vi "Index to cluster.vi"(8 "error in":errorcluster, 10 "Input Mapping Info":T1, 11 "Variant in":variant) -> (0 "error out":errorcluster, 3 "Variant out":variant)   [LabVIEW 2013]
uses:
  Channel Run Time Mapping Info.ctl
  <vilib>/Utility/VariantDataType/Type.ctl
  <vilib>/Utility/VariantDataType/VariantType.lvlib
  <vilib>/NI/Tag Bus Module Framework/root configuration/TBM configuration.lvclass
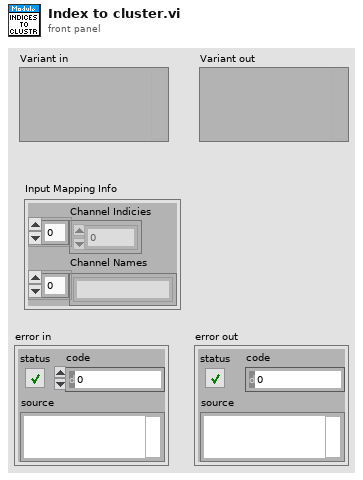
[diagram p1: front panel]
types:
  T1 = typedef "Channel Run Time Mapping Info.ctl" = cluster{"Channel Indicies":i32[], "Channel Names":string[]}
  T2 = typedef "VariantType.lvlib/Type.ctl" = enum8{"Invalid Type", "Void", "I8", "I16", "I32", "I64", "U8", "U16", "U32", "U64", "Single Float", "Double Float", "Extended Float", "Single Complex", "Double Complex", "Extended Complex", "Enum U8", "Enum U16", "Enum U32", "Enum U64", "Single Float With Unit", "Double Float With Unit", "Extended Float With Unit", "Single Complex with Unit", "Double Complex with Unit", "Extended Complex with Unit", "Boolean", "String", "Path", "Picture", "Tag", "Array", "Cluster", "Variant", "LV Variant", "Waveform", "Timestamp", "Digital Waveform", "Digital Data", "ExpressData", "Refnum", "External Data", "VI", "Poly VI", "LabVIEW Class Instance", "Fixed Point"}
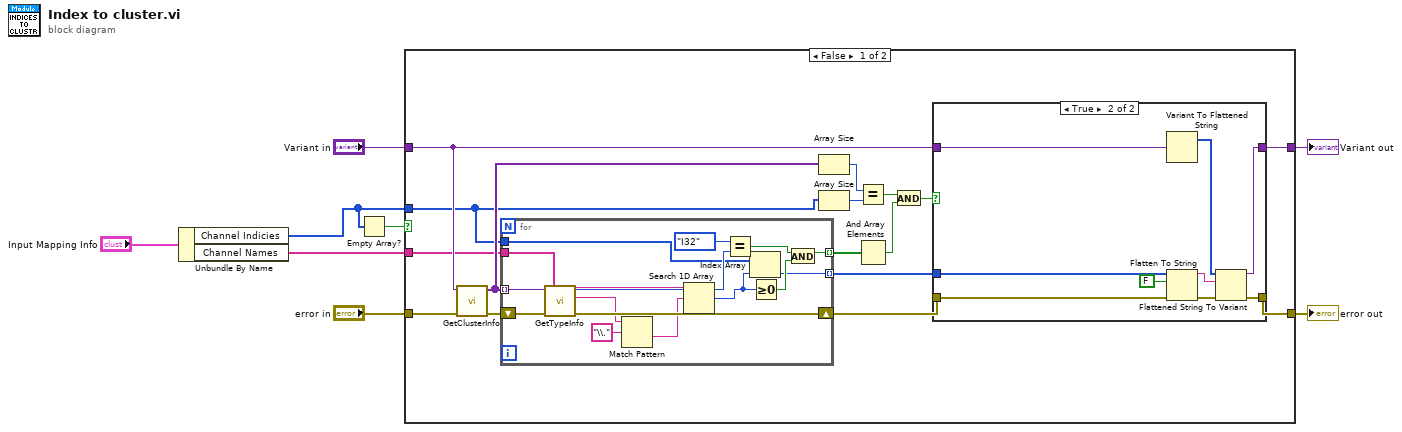
[diagram p0: block diagram]
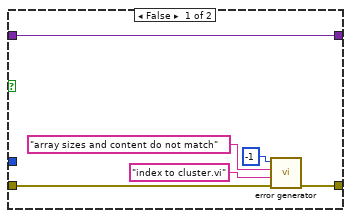
[diagram p2: hidden frame]
diagram:
  n1 = Unbundle By Name("Input Mapping Info") -> ("Channel Indicies"=w2:i32[], "Channel Names"=w1:string[])
  n2 = Empty Array?(array=w2) -> (empty?=w4:bool)
  n3 = case shown="False" w4 {
    tunnel: [w24 w56] -> w8
    tunnel: [w23 w55] -> w7
    tunnel: "error in" -> [w22 w55]
    tunnel: "Variant in" -> [w21 w56]
    tunnel: w2 -> [w10 _]
    tunnel: w1 -> [w11 _]
    frame False {
      n4 = call <vilib>:"GetClusterInfo.vi"("error in (no error)"=w22, "Variant"=w21) -> ("error out"=w17:errorcluster, "Cluster Elements"=w13:variant[])  [unwired: 8 in]
      n5 = for {
        shift-right: [w35] -> w16
        shift-left: w17 -> [w39]
        tunnel: w13 -> [w38] mode=indexing
        tunnel: [w32] -> w12 mode=indexing
        tunnel: w11 -> [w33]
        tunnel: w10 -> [w30]
        tunnel: [w28] -> w9 mode=indexing
        n6 = call <vilib>:"GetTypeInfo.vi"("error in (no error)"=w39, "Variant"=w38) -> ("error out"=w35:errorcluster, "Name"=w26:string, "Type Enum"=w37:T2)  [unwired: 5 in, 2 out]
        n7 = Match Pattern(string=w26, regular expression="\\.") -> (after substring=w27:string)  [unwired: 1 in, 3 out]
        n8 = Search 1D Array(1D array=w33, element=w27) -> (index of element=w29:i32)  [unwired: 1 in]
        n9 = Equal?(x=Type."I32", y=w37) -> (x = y?=w34:bool)
        n10 = Index Array(array=w30, index=w29) -> (element=w28:i32)
        n11 = Greater Or Equal To 0?(x=w29) -> (x >= 0?=w31:bool)
        n12 = And(x=w34, y=w31) -> (x .and. y?=w32:bool)
      }
      n13 = Array Size(array=w13) -> (size(s)=w20:i32)
      n14 = Array Size(array=w10) -> (size(s)=w19:i32)
      n15 = Equal?(x=w20, y=w19) -> (x = y?=w18:bool)
      n16 = And Array Elements(Boolean array=w12) -> (logical AND=w14:bool)
      n17 = And(x=w18, y=w14) -> (x .and. y?=w15:bool)
      n18 = case shown="True" w15 {
        tunnel: [w45 w54] -> w24
        tunnel: [w43 w53] -> w23
        tunnel: w16 -> [w44 w48]
        tunnel: w21 -> [w45 w47]
        tunnel: w9 -> [_ w46]
        frame False {
          n19 = call <vilib>:"error generator.vi"("error in"=w44, "source"="index to cluster.vi", "append error message"="array sizes and content do not match", "error code (0)"=-1) -> ("error out"=w43:errorcluster)  [unwired: 7 in]
        }
        frame True {
          n20 = Variant To Flattened String(Variant=w47) -> (1:w50:i16[])  [unwired: 1 out]
          n21 = Flatten To String(anything=w46, prepend array or string size? (T)=FALSE, error in (no error)=w48) -> (data string=w51:string, error out=w52:errorcluster)  [unwired: 1 in, 1 out]
          n22 = Flattened String To Variant(4:w52, 6:w51, 7:w50) -> (0:w53:errorcluster, 3:w54:variant)
        }
      }
    }
    frame True {
    }
  }
  "Variant out" <- w8
  "error out" <- w7
